vi "Dispense FN - ON (SubVI).vi"(0 "Signals IN":T1={"Dispense"=FALSE, "Fill"=FALSE, "Spray"=FALSE, "Drain"=TRUE, "Complete"=FALSE, "Fill Error"=FALSE, "Disp. Error"=FALSE, "Fill Timeout"=FALSE, "Disp. Timeout"=FALSE, "Purge"=TRUE}, 1 "Values IN":T3 {"Drain Time (s)" format="%.2f"; "Drain Rate (g/sec)" format="%.2f"}, 2 "Settings":T2={"ON Settings"={"Enable Dynamic Setpoint?"=TRUE, "Enable Dynamic Dispense Time?"=TRUE, "Enable Drain Rate Functions"=TRUE, "Dispense Sample Time (s)"=0.1, "Mass Average Samples"=20, "ON Timeout (sec)"=300.0, "1st Setpoint (% of Target)"=90.0, "2nd Setpoint (% of Target)"=95.0, "3rd Setpoint (% of Target)"=100.0, "Measure Dispense Delay (sec)"=10.0, "Minimum Spray Time (s)"=2.0, "Pump Reverse Time (s)"=10.0}, "OFF Settings"={"Drain Sample Time (s)"=0.1, "Drain Rate Ave Size"=100, "Drain Rate Limits (± g/sec)"=100.0, "Level Slope Range (± g/sec)"=0.05, "OFF Timeout (sec)"=300.0, "Near SP Slope Level (± g/sec)"=0.005, "Near Setpoint Threshold (%)"=99.0}, "Overshoot Settings"={"Time Limit (s)"=30.0, "Container MAX (g)"=1500.0, "Max FILL Slope (+/- g/sec)"=100.0, "% Overshot to Enable (>)"=3.0}, "FILL Timeout (s)"=300.0, "Full \nSettle Time (s)"=30.0, "Pre-Hydrate \nSpray Time (s)"=0.0, "Pre-Hydrate \nWait Time (s)"=10.0, "m Value "=1.0, "b Value"=0.0, "Enable Overshoot Adjust?"=FALSE} {"ON Settings"."Pump Reverse Time (s)" min=0.0 max=60.0; "OFF Settings"."Near SP Slope Level (± g/sec)" format="%.3g"; "OFF Settings"."Level Slope Range (± g/sec)" format="%.3g"}, 3 "Main Concentration Setpoint (%)":dbl, 4 "Measured Mass (g)":dbl, 5 "State Change?":bool, 7 "Main Case Change?":bool) -> (14 "Signals OUT":T1={"Dispense"=FALSE, "Fill"=FALSE, "Spray"=FALSE, "Drain"=TRUE, "Complete"=FALSE, "Fill Error"=FALSE, "Disp. Error"=FALSE, "Fill Timeout"=FALSE, "Disp. Timeout"=FALSE, "Purge"=TRUE}, 15 "Values OUT":T3 {"Drain Time (s)" format="%.2f"; "Drain Rate (g/sec)" format="%.2f"}, 17 "Spray Count":i32, 19 "OFF Signal":bool)   [LabVIEW 2011]
uses:
  <vilib>/ptbypt/NI_PtbyPt.lvlib
panel:
  # "ONLY ADJUST\nBOLD VALUES!"
  # "Corrected Mass = SDC Mass * m + b"
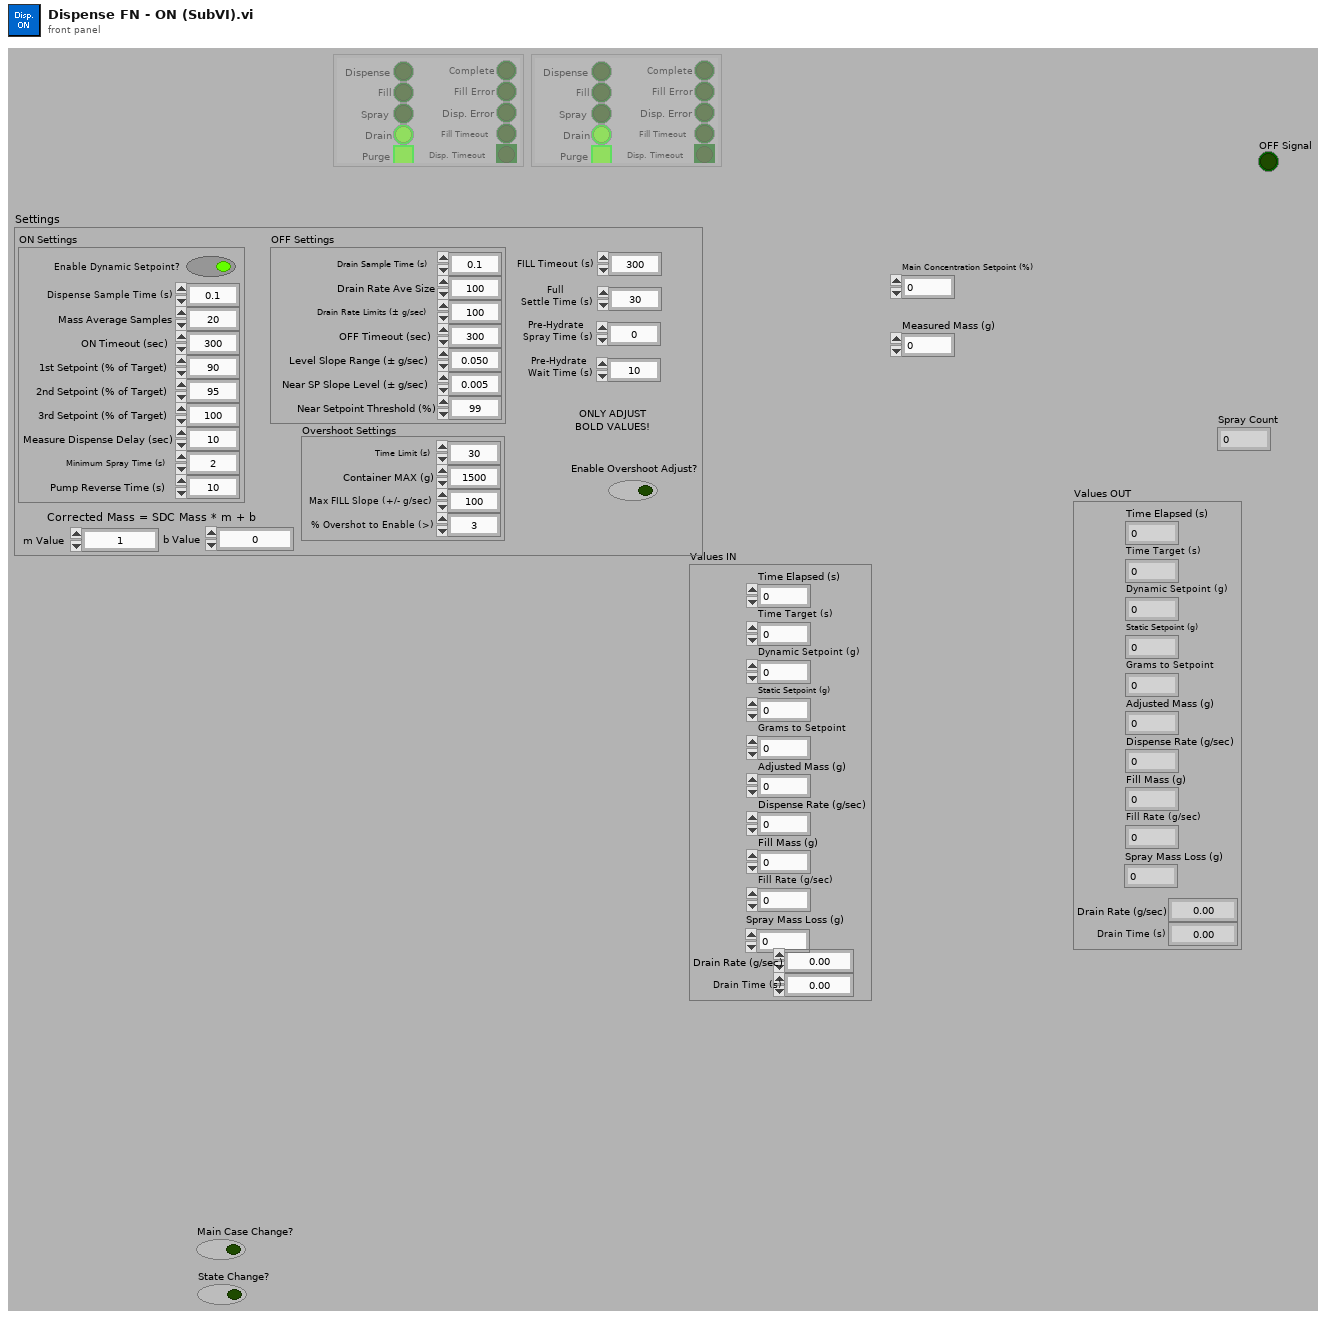
[diagram p1: front panel]
types:
  T1 = cluster{"Dispense":bool, "Fill":bool, "Spray":bool, "Drain":bool, "Complete":bool, "Fill Error":bool, "Disp. Error":bool, "Fill Timeout":bool, "Disp. Timeout":bool, "Purge":bool}
  T2 = cluster{"ON Settings":cluster{"Enable Dynamic Setpoint?":bool, "Enable Dynamic Dispense Time?":bool, "Enable Drain Rate Functions":bool, "Dispense Sample Time (s)":dbl, "Mass Average Samples":i32, "ON Timeout (sec)":dbl, "1st Setpoint (% of Target)":dbl, "2nd Setpoint (% of Target)":dbl, "3rd Setpoint (% of Target)":dbl, "Measure Dispense Delay (sec)":dbl, "Minimum Spray Time (s)":dbl, "Pump Reverse Time (s)":dbl}, "OFF Settings":cluster{"Drain Sample Time (s)":dbl, "Drain Rate Ave Size":i32, "Drain Rate Limits (± g/sec)":dbl, "Level Slope Range (± g/sec)":dbl, "OFF Timeout (sec)":dbl, "Near SP Slope Level (± g/sec)":dbl, "Near Setpoint Threshold (%)":dbl}, "Overshoot Settings":cluster{"Time Limit (s)":dbl, "Container MAX (g)":dbl, "Max FILL Slope (+/- g/sec)":dbl, "% Overshot to Enable (>)":dbl}, "FILL Timeout (s)":dbl, "Full \nSettle Time (s)":dbl, "Pre-Hydrate \nSpray Time (s)":dbl, "Pre-Hydrate \nWait Time (s)":dbl, "m Value ":dbl, "b Value":dbl, "Enable Overshoot Adjust?":bool}
  T3 = cluster{"Time Elapsed (s)":dbl, "Time Target (s)":dbl, "Dynamic Setpoint (g)":dbl, "Static Setpoint (g)":dbl, "Grams to Setpoint":dbl, "Adjusted Mass (g)":dbl, "Dispense Rate (g/sec)":dbl, "Fill Mass (g)":dbl, "Fill Rate (g/sec)":dbl, "Spray Mass Loss (g)":dbl, "Drain Rate (g/sec)":dbl, "Drain Time (s)":dbl}
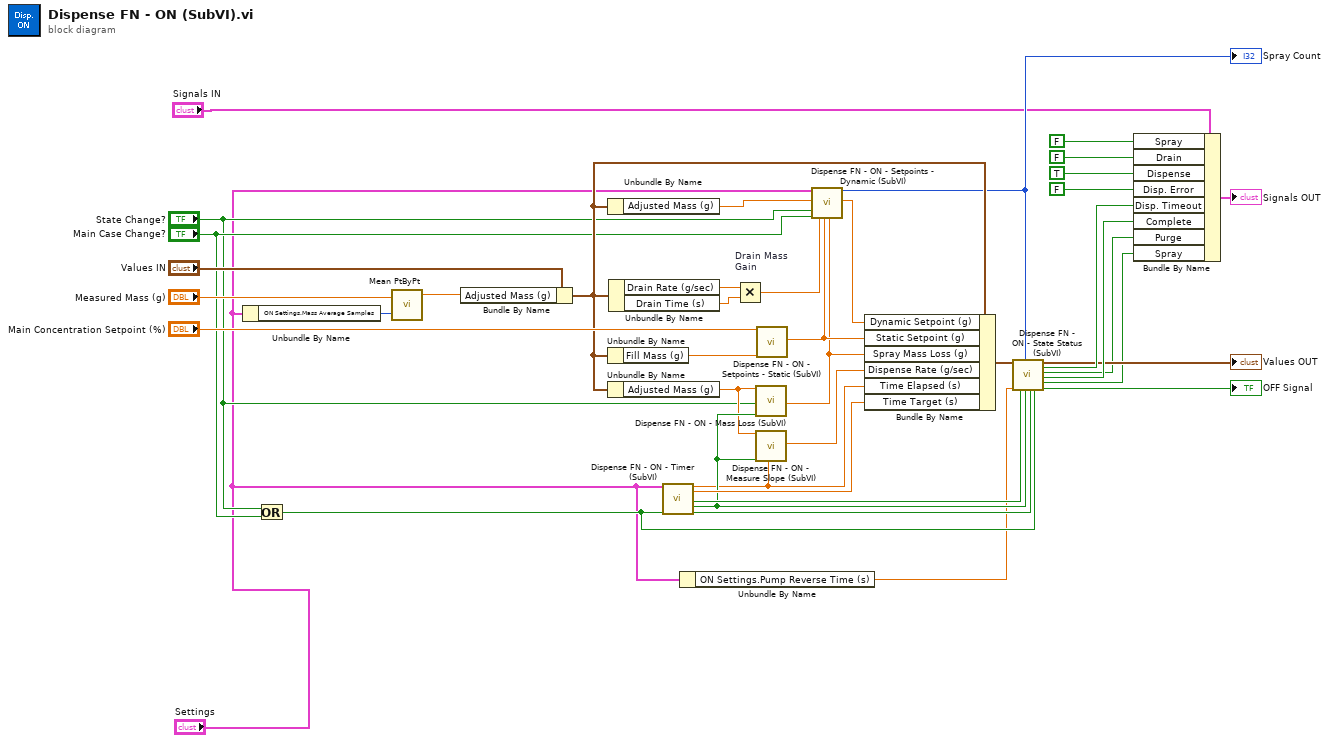
[diagram p0: block diagram]
diagram:
  n1 = Unbundle By Name("Settings") -> ("ON Settings.Mass Average Samples"=w27:i32)
  n2 = Or(x="State Change?", y="Main Case Change?") -> (x .or. y?=w7:bool)
  n3 = call <vilib>:"Mean PtByPt.vi"("x"="Measured Mass (g)", "sample length"=w27) -> ("mean"=w30:dbl)  [unwired: 1 in, 2 out]
  n4 = Bundle By Name(cluster="Values IN", "Adjusted Mass (g)"=w30) -> (w16:T3)
  n5 = Unbundle By Name(w16) -> ("Adjusted Mass (g)"=w29:dbl)
  n6 = Unbundle By Name(w16) -> ("Fill Mass (g)"=w36:dbl)
  n7 = Unbundle By Name(w16) -> ("Adjusted Mass (g)"=w18:dbl)
  n8 = Unbundle By Name(w16) -> ("Drain Rate (g/sec)"=w35:dbl, "Drain Time (s)"=w34:dbl)
  n9 = call "Dispense FN - ON - Timer (SubVI).vi"("Settings"="Settings", "Reset"=w7) -> ("Elapsed Time (s)"=w17:dbl, "ON Timeout (s)"=w26:dbl, "Min Spray Complete?"=w22:bool, "Measure Delay Complete?"=w21:bool, "Max Spray Complete?"=w20:bool)  [unwired: 13 in]
  n10 = Unbundle By Name("Settings") -> ("ON Settings.Pump Reverse Time (s)"=w1:dbl)
  n11 = Multiply "Drain Mass\nGain"(x=w35, y=w34) -> (x*y=w33:dbl)
  n12 = call "Dispense FN - ON - Mass Loss (SubVI).vi"("Measured Mass (g)"=w18, "State Change?"="State Change?", "Measure Delay Complete?"=w21) -> ("Dispense Mass Loss"=w31:dbl)  [unwired: 16 in]
  n13 = call "Dispense FN - ON - Measure Slope (SubVI).vi"("Measured Mass (g)"=w18, "Measure Delay Complete?"=w21, "Elapsed Time (s)"=w17) -> ("Ave. Slope (g/sec)"=w19:dbl)  [unwired: 16 in]
  n14 = call "Dispense FN - ON - Setpoints - Static (SubVI).vi"("Main Concentration Setpoint (%)"="Main Concentration Setpoint (%)", "Fill Mass (g)"=w36) -> ("Static Setpoint (g)"=w32:dbl)  [unwired: 17 in]
  n15 = call "Dispense FN - ON - Setpoints - Dynamic (SubVI).vi"("Settings"="Settings", "Measured Mass (g)"=w29, "State Change?"="State Change?", "Main Case Change?"="Main Case Change?", "Drain Mass Gain (g)"=w33, "Static Setpoint (g)"=w32, "Spray Mass Loss (g)"=w31) -> ("Spray Count"=w13:i32, "Dynamic Setpoint (g)"=w38:dbl)  [unwired: 11 in]
  "Spray Count" <- w13
  n16 = Bundle By Name(cluster=w16, "Dynamic Setpoint (g)"=w38, "Static Setpoint (g)"=w32, "Spray Mass Loss (g)"=w31, "Dispense Rate (g/sec)"=w19, "Time Elapsed (s)"=w17, "Time Target (s)"=w26) -> (w12:T3)
  n17 = call "Dispense FN - ON - State Status (SubVI).vi"("Values IN"=w12, "Reverse/Purge Time (s)"=w1, "Min Spray Complete?"=w22, "Spray Count"=w13, "Measure Delay Complete?"=w21, "Max Spray Complete?"=w20, "Reset?"=w7) -> ("Values OUT"=→"Values OUT":T3, "Dispense Timeout?"=w25:bool, "Purge Signal"=w4:bool, "Complete"=w24:bool, "Spray Signal"=w3:bool, "OFF Signal"=→"OFF Signal":bool)  [unwired: 5 in, 2 out]
  n18 = Bundle By Name(cluster="Signals IN", "Spray"=FALSE, "Drain"=FALSE, "Dispense"=TRUE, "Disp. Error"=FALSE ("Dispense Error"), "Disp. Timeout"=w25, "Complete"=w24, "Purge"=w4, "Spray"=w3) -> (→"Signals OUT":T1)
